vi "My OWn PID.vi"(8 "Current Input":dbl, 11 "Wanted End":dbl) -> (3 "Output":dbl)   [LabVIEW 2017]
panel:
  in  "Encoders (t) gyro (f)":bool
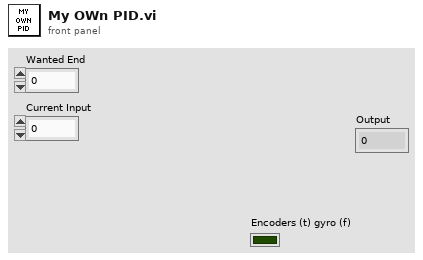
[diagram p1: front panel]
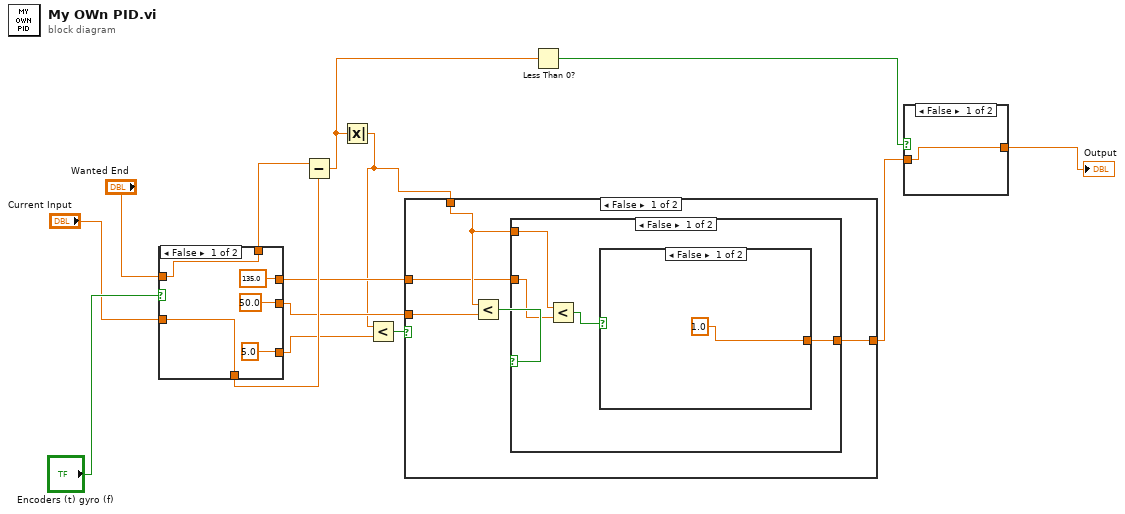
[diagram p0: block diagram]
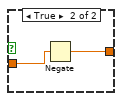
[diagram p2: hidden frame]
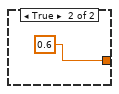
[diagram p3: hidden frame]
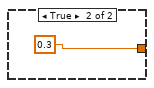
[diagram p4: hidden frame]
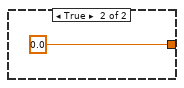
[diagram p5: hidden frame]
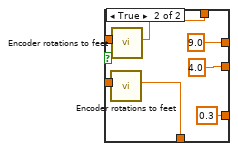
[diagram p6: hidden frame]
diagram:
  n1 = case shown="False" "Encoders (t) gyro (f)" {
    tunnel: "Wanted End" -> [w19 w26]
    tunnel: "Current Input" -> [w18 w25]
    tunnel: [w19 w24] -> w11
    tunnel: [w18 w23] -> w10
    tunnel: [135.0 9.0] -> w6
    tunnel: [50.0 4.0] -> w7
    tunnel: [5.0 0.3] -> w8
    frame False {
    }
    frame True {
      n2 = call "Encoder rotations to feet.vi"("Encoder Rotations"=w25) -> ("Feet"=w23:dbl)  [unwired: 10 in]
      n3 = call "Encoder rotations to feet.vi"("Encoder Rotations"=w26) -> ("Feet"=w24:dbl)  [unwired: 10 in]
    }
  }
  n4 = Subtract(x=w11, y=w10) -> (x-y=w4:dbl)
  n5 = Absolute Value(x=w4) -> (abs(x)=w5:dbl)
  n6 = Less?(x=w5, y=w8) -> (x < y?=w9:bool)
  n7 = case shown="False" w9 {
    tunnel: w5 -> [w28 _]
    tunnel: [w29 0.0] -> w2
    tunnel: w7 -> [w31 _]
    tunnel: w6 -> [w27 _]
    frame False {
      n8 = Less?(x=w28, y=w31) -> (x < y?=w30:bool)
      n9 = case shown="False" w30 {
        tunnel: [w33 0.3] -> w29
        tunnel: w28 -> [w35 _]
        tunnel: w27 -> [w34 _]
        frame False {
          n10 = Less?(x=w35, y=w34) -> (x < y?=w32:bool)
          n11 = case shown="False" w32 {
            tunnel: [1.0 0.6] -> w33
            frame False {
            }
            frame True {
            }
          }
        }
        frame True {
        }
      }
    }
    frame True {
    }
  }
  n12 = Less Than 0?(x=w4) -> (x < 0?=w3:bool)
  n13 = case shown="False" w3 {
    tunnel: w2 -> [w40 w42]
    tunnel: [w40 w41] -> w1
    frame False {
    }
    frame True {
      n14 = Negate(x=w42) -> (-x=w41:dbl)
    }
  }
  "Output" <- w1
